vi "FlakyDelegate-dotNETeventRelay.vi"(4 "Relayed event":refnum<user-event>, 5 "Event Data":cluster{"sender":refnum<k24>, "e":refnum<k24>}, 6 "Control Ref":refnum<k24>, 7 "Event Common Data":T1) -> ()   [LabVIEW 2012]
uses:
  System.Windows.Forms
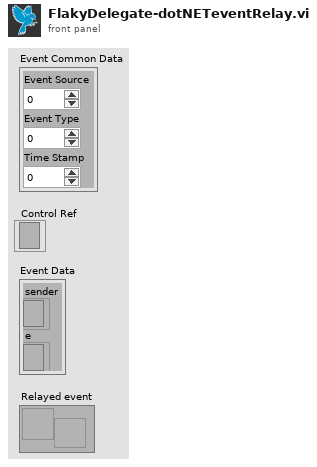
[diagram p1: front panel]
types:
  T1 = cluster{"Event Source":i32, "Event Type":u32, "Time Stamp":u32}
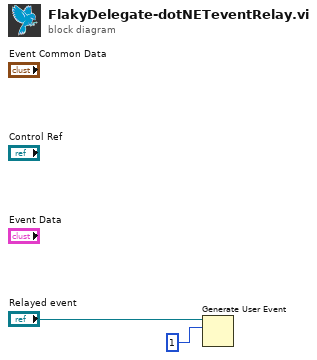
[diagram p0: block diagram]
diagram:
  n1 = Generate User Event(user event="Relayed event", event data cluster=1 ("event data")) -> ()  [unwired: 1 in, 2 out]
